vi "ziExample-HF2-PLL.vi"() -> ()   [LabVIEW 2009]
doc: "Control a Zurich instrument device via the LabOne Labview API. \nRequirements: Zurich Instruments HF2.\nThis example implements a simple PLL in LabVIEW.\n\n© Zurich Instruments AG, www.zhinst.com"
uses:
  <instrlib>/Zurich Instruments LabOne/Public/Utility/ziTicksToS_single.vi
  <instrlib>/Zurich Instruments LabOne/Public/Configure/ziGetValueDemodSampleEx.vi
  <instrlib>/Zurich Instruments LabOne/Zurich Instruments LabOne.lvlib
panel:
  out "Error Out":errorcluster
  out "output cluster":cluster{dbl[], dbl[]}
  out "Selected Device":string
  in  "Address":string="DEV"
  in  "DefaultSettings":bool
  in  "RefPhase":dbl=36.0 caption="Ref Phase (deg)"
  out "Error":dbl=0.0011898289611309565 format="%+8.5f°"
  out "Frequency":ext=1839836.4116389132 format="%_9pHz"
  out "Rate":dbl=94.24546185775438 format="%5.0pHz"
  in  "Gain":dbl(slide)=1.0 scale=0.1..1000.0 scale format="%#_6p"
  out "Phase":dbl=89.99881017103887 format="%+9.4g°"
  in  "CenterFreq":dbl=1838000.0 caption="Center Freq" format="%_6pHz"
  in  "SendFreq":bool
  out "Amplitude":dbl(graph)=1.0771498465688651
  out "Frequency":dbl(graph)
  in  "EnablePLL":bool=TRUE caption="Enable PLL"
  out "Timeconstant":dbl format="%#_3ps"
  out "Y":dbl=1.0771498463366156 format="%+_6pVrms"
  out "Amp":dbl=1.0771498465688651 format="%_6pVrms"
  out "X":dbl=2.2368173693618797e-05 format="%+_6pVrms"
  in  "Filter Order":u16=4
  in  "stop":bool=TRUE
  in  "Bandwidth":dbl=100.0
  # "Notes:\nCRYSTAL, HC-49/U, 1.8432MHZ; Frequenz, A\nIf signal very unstable: change gain (value of 1000 shows good stability), \nor check if you have the right peak (use set frequency and use the sweeper to find the right peak)\n\nThis PLL implmentation is very slow (more than 1000 times slower) compared to the PLL option that is \navailable for Zurich Instruments Lock-in Amplifiers. The PLL Option runs inside the instrument itself."
  # "Tested Instruments:\n- HF2LI"
  # "Filter Settings"
  # "PLL Settings"
  # "PLL Monitor"
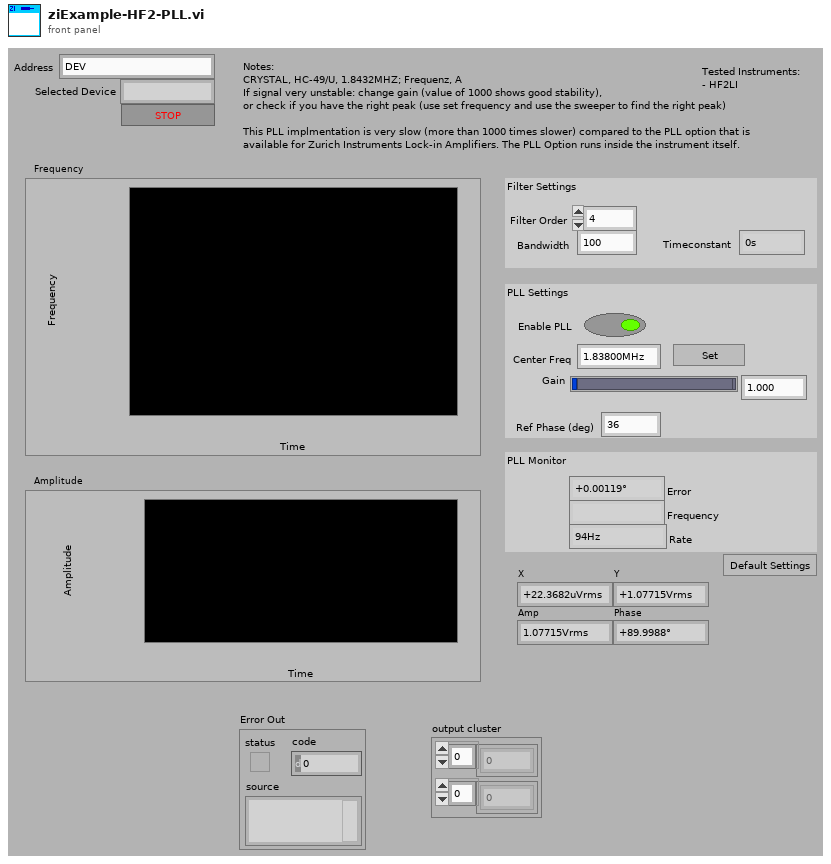
[diagram p1: front panel]
types:
  T1 = typedef "Zurich Instruments LabOne.lvlib/ziTypeHandle.ctl" = cluster{"handleValid":bool, "Conn":u64, "Path Prefix":string, "Handle":u64, "Connected":bool, "Clockbase(s)":dbl}
  T2 = typedef "Zurich Instruments LabOne.lvlib/ziTypeDemodSampleSingle.ctl" = cluster{"Timestamps (ticks)":u64, "X (Vrms)":dbl, "Y (Vrms)":dbl, "Osc Phase (deg)":dbl, "Freq (Hz)":dbl, "DIO":u32, "AuxIn0 (V)":dbl, "AuxIn1 (V)":dbl, "Trigger":u32}
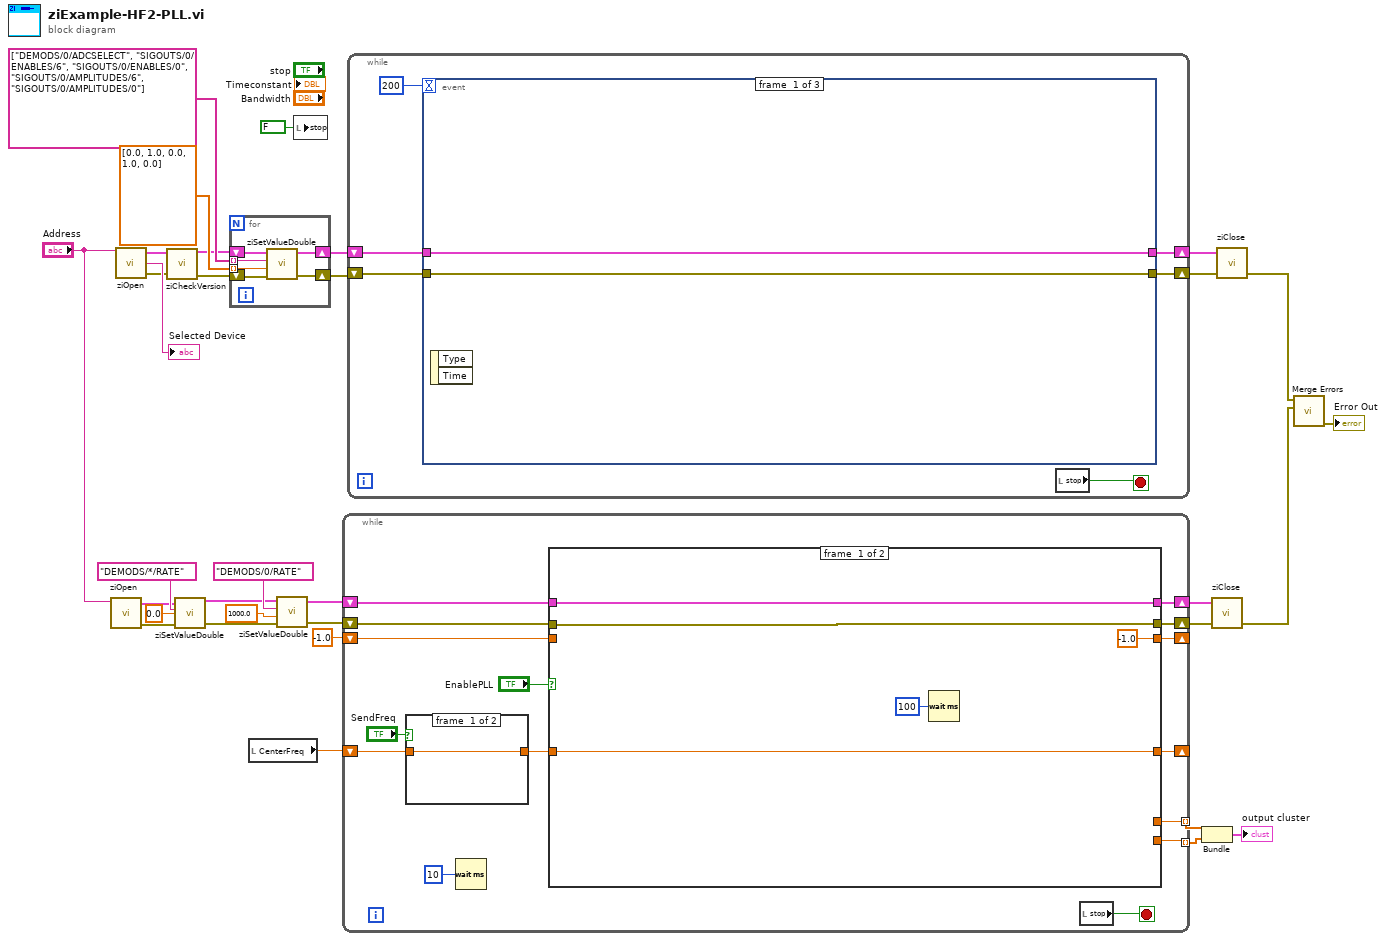
[diagram p0: block diagram]
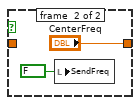
[diagram p2: hidden frame]
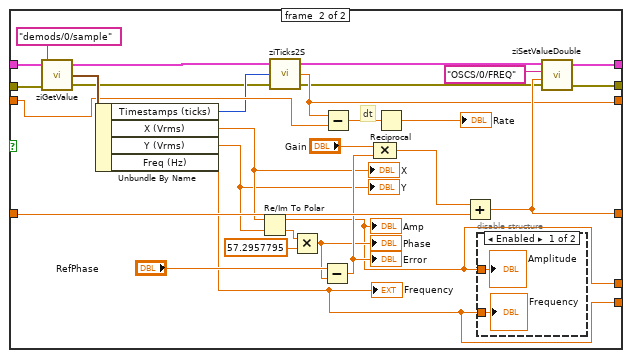
[diagram p3: hidden frame]
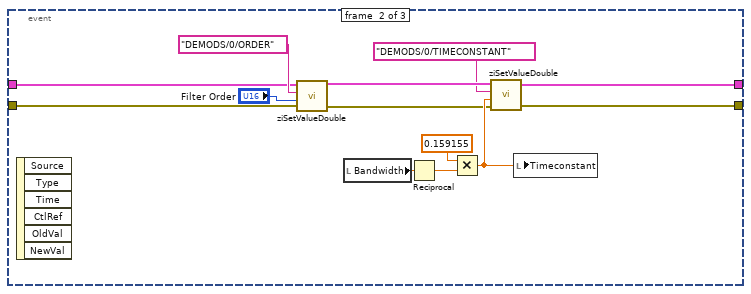
[diagram p5: hidden frame]
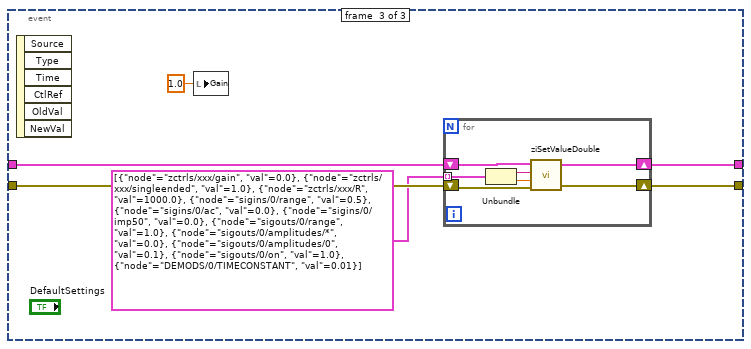
[diagram p6: hidden frame]
diagram:
  n1 = call <instrlib>:"ziOpen.vi"("Address"="Address") -> ("Error Out"=w21:errorcluster, "HandleOut"=w20:T1)  [unwired: 1 in, 3 out]
  n2 = call <instrlib>:"ziOpen.vi"("Address"="Address") -> ("Error Out"=w3:errorcluster, "Selected Device"=→"Selected Device":string, "HandleOut"=w4:T1)  [unwired: 1 in, 2 out]
  n3 = call <instrlib>:"ziCheckVersion.vi"("Handle In"=w4, "Error In"=w3) -> ("Handle Out"=w2:T1, "Error Out"=w1:errorcluster)  [unwired: 11 in, 1 out]
  n4 = call <instrlib>:"ziSetValueDouble.vi"("Error In"=w21, "Value"=0.0, "Path"="DEMODS/*/RATE" ("Path (\"/\")"), "Handle In"=w20) -> ("Error Out"=w26:errorcluster, "Handle Out"=w25:T1)  [unwired: 1 out]
  n5 = for {
    tunnel: string[] ["DEMODS/0/ADCSELECT", "SIGOUTS/0/ENABLES/6", "SIGOUTS/0/ENABLES/0", "SIGOUTS/0/AMPLITUDES/6", "SIGOUTS/0/AMPLITUDES/0"] -> [w36] mode=indexing
    tunnel: dbl[] [0.0, 1.0, 0.0, 1.0, 0.0] -> [w35] mode=indexing
    shift-right: [w38] -> w14
    shift-left: w2 -> [w39]
    shift-right: [w37] -> w13
    shift-left: w1 -> [w34]
    n6 = call <instrlib>:"ziSetValueDouble.vi"("Error In"=w34, "Value"=w35, "Path"=w36, "Handle In"=w39) -> ("Error Out"=w37:errorcluster, "Handle Out"=w38:T1)  [unwired: 1 out]
  }
  n7 = local read "CenterFreq"() -> (w22:dbl)
  n8 = call <instrlib>:"ziSetValueDouble.vi"("Error In"=w26, "Value"=1000.0, "Path"="DEMODS/0/RATE" ("Path (\"/\")"), "Handle In"=w25) -> ("Error Out"=w19:errorcluster, "Handle Out"=w18:T1)  [unwired: 1 out]
  n9 = local write "stop"(FALSE ("stop")) -> ()
  n10 = while {
    shift-right: [w51] -> _
    shift-left: w22 -> [w49]
    shift-right: [w54] -> w28
    shift-left: w18 -> [w46]
    shift-right: [w53] -> w27
    shift-left: w19 -> [w47]
    shift-right: [w43] -> _
    shift-left: -1.0 ("Timestamps (s)") -> [w44]
    tunnel: [w41] -> w9 mode=indexing
    tunnel: [w40] -> w10 mode=indexing
    stop <- w52 stop-if-true
    n11 = case shown="True" "SendFreq" {
      tunnel: w49 -> [w55 _]
      tunnel: [w55 "CenterFreq"] -> w48
      frame #0 {
      }
      frame #1 {
        n12 = local write "SendFreq"(FALSE ("Set Frequency (PLL off)")) -> ()
      }
    }
    n13 = Wait (ms)(milliseconds to wait=u32 10) -> ()  [unwired: 1 out]
    n14 = case shown="True" "EnablePLL" {
      tunnel: w46 -> [w62 w83]
      tunnel: w47 -> [w61 w82]
      tunnel: [w62 w88] -> w54
      tunnel: [w61 w89] -> w53
      tunnel: w48 -> [w60 w91]
      tunnel: [w60 w87] -> w51
      tunnel: w44 -> [_ w76]
      tunnel: [-1.0 ("Timestamps (s)") w69] -> w43
      tunnel: [_ w64] -> w40
      tunnel: [_ w63] -> w41
      frame #0 {
        n15 = Wait (ms)(milliseconds to wait=u32 100) -> ()  [unwired: 1 out]
      }
      frame #1 {
        # "dt"
        n16 = call-poly <instrlib>:"ziGetValue.vi"("error in"=w82, "Path"="demods/0/sample" ("Path ()"), "Handle In"=w83) -> ("error out"=w66:errorcluster, "Demod Sample Out"=w79:T2, "Handle Out"=w68:T1)
        n17 = Unbundle By Name(w79) -> ("Timestamps (ticks)"=w70:u64, "X (Vrms)"=w78:dbl, "Y (Vrms)"=w77:dbl, "Freq (Hz)"=w63:dbl)
        "X" <- w78
        "Y" <- w77
        "Frequency" <- w63
        n18 = Re/Im To Polar(2:w77, 3:w78) -> (0:w86:dbl, 1:w64:dbl)
        "Amp" <- w64
        n19 = call-poly <instrlib>:"ziTicks2S.vi"("Error In"=w66, "Timestamp(ticks)"=w70, "Handle In"=w68) -> ("Error Out"=w65:errorcluster, "Timestamp(s)"=w69:dbl, "Handle Out"=w67:T1)
        n20 = Multiply(x=w86, y=57.2957795) -> (x*y=w72:dbl)
        "Phase" <- w72
        n21 = Subtract(x="RefPhase", y=w72) -> (x-y=w80:dbl)
        "Error" <- w80
        n22 = Subtract(x=w69, y=w76) -> (x-y=w71:dbl)
        n23 = Compound Arithmetic op=MULTIPLY("Gain", w80) -> (w73:dbl)
        n24 = Reciprocal(x=w71) -> (1/x=→"Rate":dbl)
        n25 = Add(x=w73, y=w91) -> (x+y=w87:dbl)
        n26 = disable-structure shown="Enabled" {
          disable-tunnel: w63 -> [w93 _]
          disable-tunnel: w64 -> [w92 _]
          frame #0 {
            "Frequency" <- w93
            "Amplitude" <- w92
          }
          frame #1 {
          }
        }
        n27 = call <instrlib>:"ziSetValueDouble.vi"("Error In"=w65, "Value"=w87, "Path"="OSCS/0/FREQ" ("name (unnamed)"), "Handle In"=w67) -> ("Error Out"=w89:errorcluster, "Handle Out"=w88:T1)  [unwired: 1 out]
      }
    }
    n28 = local read "stop"() -> (w52:bool)
  }
  n29 = while {
    shift-right: [w95] -> w30
    shift-left: w14 -> [w97]
    shift-right: [w94] -> w29
    shift-left: w13 -> [w96]
    stop <- w98 stop-if-true
    n30 = event shown="[1] \"Bandwidth\", \"Filter Order\": Value Change" {
      selector: _ -> [_ _ _]
      dyn-events: _ -> [_ _ _]
      timeout: 200 -> [_ _ _]
      tunnel: w97 -> [w101 w103 w118]
      tunnel: w96 -> [w100 w102 w117]
      tunnel: [w101 w105 w120] -> w95
      tunnel: [w100 w104 w119] -> w94
      event #0 {
        n31 = event-data() -> ()  [unwired: 3 out]
      }
      event #1 {
        n32 = event-data() -> ()  [unwired: 7 out]
        n33 = call <instrlib>:"ziSetValueDouble.vi"("Error In"=w102, "Value"="Filter Order", "Path"="DEMODS/0/ORDER" ("name (unnamed)"), "Handle In"=w103) -> ("Error Out"=w111:errorcluster, "Handle Out"=w110:T1)  [unwired: 1 out]
        n34 = local read "Bandwidth"() -> (w109:dbl)
        n35 = Reciprocal(x=w109) -> (1/x=w108:dbl)
        n36 = Multiply(x=0.159155 ("y"), y=w108) -> (x*y=w114:dbl)
        n37 = call <instrlib>:"ziSetValueDouble.vi"("Error In"=w111, "Value"=w114, "Path"="DEMODS/0/TIMECONSTANT" ("name (unnamed)"), "Handle In"=w110) -> ("Error Out"=w104:errorcluster, "Handle Out"=w105:T1)  [unwired: 1 out]
        n38 = local write "Timeconstant"(w114) -> ()
      }
      event #2 {
        n39 = event-data() -> ()  [unwired: 7 out]
        n40 = local write "Gain"(1.0 ("Gain")) -> ()
        n41 = for {
          tunnel: cluster{"node":string, "val":dbl}[] [{"node"="zctrls/xxx/gain", "val"=0.0}, {"node"="zctrls/xxx/singleended", "val"=1.0}, {"node"="zctrls/xxx/R", "val"=1000.0}, {"node"="sigins/0/range", "val"=0.5}, {"node"="sigins/0/ac", "val"=0.0}, {"node"="sigins/0/imp50", "val"=0.0}, {"node"="sigouts/0/range", "val"=1.0}, {"node"="sigouts/0/amplitudes/*", "val"=0.0}, {"node"="sigouts/0/amplitudes/0", "val"=0.1}, {"node"="sigouts/0/on", "val"=1.0}, {"node"="DEMODS/0/TIMECONSTANT", "val"=0.01}] -> [w123] mode=indexing
          shift-right: [w126] -> w120
          shift-left: w118 -> [w127]
          shift-right: [w125] -> w119
          shift-left: w117 -> [w124]
          n42 = Unbundle(w123) -> ("node"=w122:string, "val"=w121:dbl)
          n43 = call <instrlib>:"ziSetValueDouble.vi"("Error In"=w124, "Value"=w121, "Path"=w122, "Handle In"=w127) -> ("Error Out"=w125:errorcluster, "Handle Out"=w126:T1)  [unwired: 1 out]
        }
      }
    }
    n44 = local read "stop"() -> (w98:bool)
  }
  n45 = Bundle(w10, w9) -> (→"output cluster":cluster{dbl[], dbl[]})  [unwired: 1 in]
  n46 = call <instrlib>:"ziClose.vi"("Error In"=w27, "Handle In"=w28) -> ("Error Out"=w6:errorcluster)  [unwired: 3 out]
  n47 = call <instrlib>:"ziClose.vi"("Error In"=w29, "Handle In"=w30) -> ("Error Out"=w7:errorcluster)  [unwired: 3 out]
  n48 = call <vilib>:"Merge Errors.vi"("error in 2 (no error)"=w6, "error in 1 (no error)"=w7) -> ("error out"=→"Error Out":errorcluster)  [unwired: 5 in]
